vi "PSUController_GCFS.vi"(3 "error in (no error)":errorcluster, 4 "VISA.PSU":refnum<visa-resource-name>, 5 "Output":string, 6 "PSU.Connected":bool) -> (0 "error out":errorcluster, 1 "Valid?":bool)   [LabVIEW 2024]
uses:
  acdbe4be-fc26-43bf-b7cf-514e7f30e473.vi
  <vilib>/regexp/Match Regular Expression.xnode
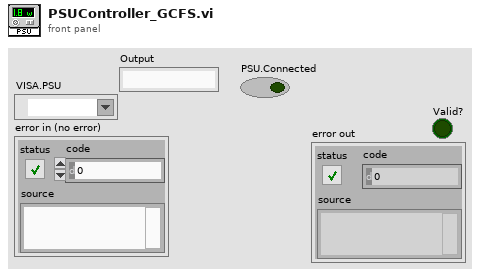
[diagram p1: front panel]
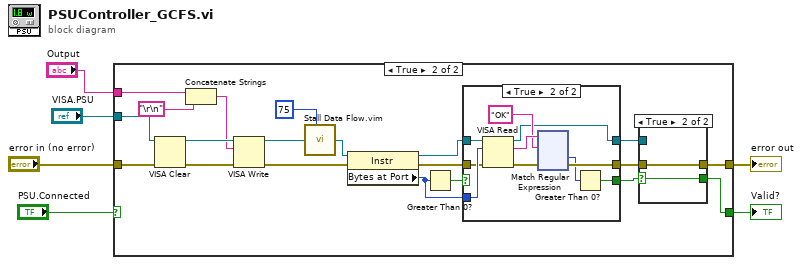
[diagram p0: block diagram]
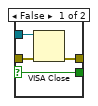
[diagram p3: hidden frame]
diagram:
  n1 = case shown="True" "PSU.Connected" {
    selector: "PSU.Connected" -> [w8 _]
    tunnel: [w7 w24] -> w4
    tunnel: [w8 w23] -> w3
    tunnel: "VISA.PSU" -> [_ w22]
    tunnel: "error in (no error)" -> [w7 w21]
    tunnel: "Output" -> [_ w9]
    frame False {
    }
    frame True {
      n2 = VISA Clear(VISA resource name=w22, error in (no error)=w21) -> (VISA resource name out=w28:refnum<visa-resource-name>, error out=w27:errorcluster)
      n3 = Concatenate Strings(w9, "\r\n") -> (w11:string)
      n4 = VISA Write(VISA resource name=w28, write buffer=w11, error in (no error)=w27) -> (VISA resource name out=w26:refnum<visa-resource-name>, error out=w25:errorcluster)  [unwired: 1 out]
      n5 = call "Stall Data Flow.vim"("value in"=w26, "milliseconds to wait"=u32 75) -> ("value out"=w20:refnum<visa-resource-name>)  [unwired: 1 out]
      n6 = property class="Instr"(reference=w20, error in=w25) -> (reference out=w17:refnum<visa-resource-name>, error out=w16:errorcluster, "Bytes at Port"=w18:u32)
      n7 = Greater Than 0?(x=w18) -> (x > 0?=w19:bool)
      n8 = case shown="True" w19 {
        selector: w19 -> [w36 _]
        tunnel: w18 -> [_ w47]
        tunnel: w16 -> [w37 w46]
        tunnel: [w37 w41] -> w13
        tunnel: w17 -> [w35 w45]
        tunnel: [w36 w39] -> w14
        tunnel: [w35 w38] -> w12
        frame False {
        }
        frame True {
          n9 = VISA Read(VISA resource name=w45, byte count=w47, error in (no error)=w46) -> (VISA resource name out=w38:refnum<visa-resource-name>, read buffer=w44:string, error out=w43:errorcluster)  [unwired: 1 out]
          n10 = xnode "Match Regular Expression"("input string"=w44, "regular expression"="OK", "error in"=w43) -> ("offset past match"=w40:i32, "error out"=w41:errorcluster)  [unwired: 3 in, 3 out]
          n11 = Greater Than 0?(x=w40) -> (x > 0?=w39:bool)
        }
      }
      n12 = case shown="True" w14 {
        selector: w14 -> [w32 w33]
        tunnel: [w29 w34] -> w24
        tunnel: w13 -> [w30 w34]
        tunnel: [w32 w33] -> w23
        tunnel: w12 -> [w31 _]
        frame False {
          n13 = VISA Close(VISA resource name=w31, error in (no error)=w30) -> (error out=w29:errorcluster)
        }
        frame True {
        }
      }
    }
  }
  "error out" <- w4
  "Valid?" <- w3
